vi "Report_Broken_VI.vi"(7 "before build?":bool=TRUE, 8 "error in (no error)":errorcluster, 10 "vi path":path, 11 "Build in":refnum<class "AB_Build.lvclass">) -> (0 "error out":errorcluster, 3 "Build out":refnum<class "AB_Build.lvclass">)   [LabVIEW 2020, in "AB_Build.lvclass"]
uses:
  <vilib>/AppBuilder/AB_Classes/Build/AB_Build.lvclass
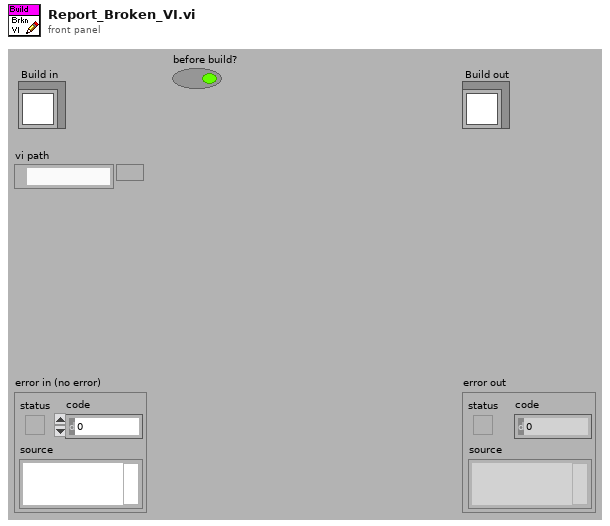
[diagram p1: front panel]
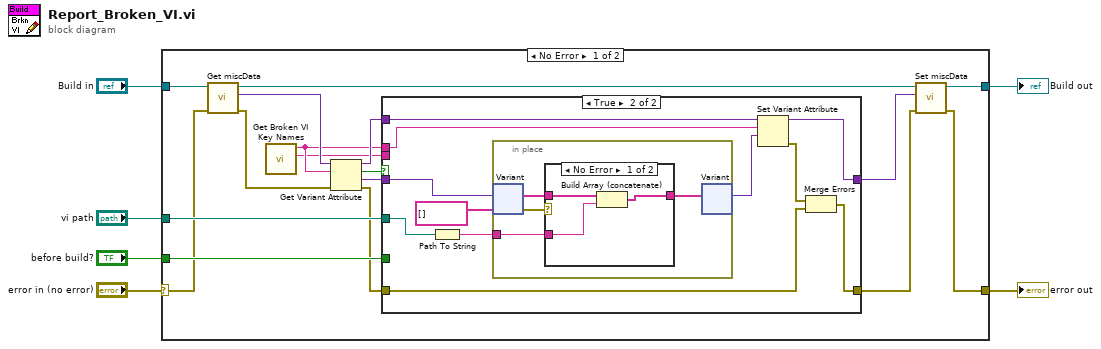
[diagram p0: block diagram]
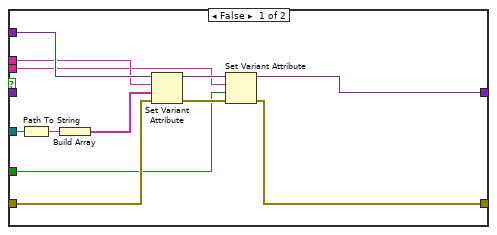
[diagram p2: hidden frame]
diagram:
  n1 = case shown="No Error" "error in (no error)" {
    selector: "error in (no error)" -> [w18 w56]
    tunnel: "Build in" -> [w23 w55]
    tunnel: [w21 w55] -> w5
    tunnel: [w11 w56] -> w4
    tunnel: "vi path" -> [w20 _]
    tunnel: "before build?" -> [w19 _]
    frame No Error {
      n2 = call-dynamic "Get miscData.vi"("error in (no error)"=w18, "AB_Build in"=w23) -> ("error out"=w15:errorcluster, "eng_miscData"=w17:variant, "AB_Build out"=w22:refnum<class "AB_Build.lvclass">)  [unwired: 7 in]
      n3 = call <vilib>:"Get Broken VI Key Names.vi"() -> ("Before Build Key"=w7:string, "Broken VIs List Key"=w8:string)  [unwired: 10 in]
      n4 = Get Variant Attribute(Variant=w17, name=w8, error in=w15) -> (duplicate Variant=w9:variant, found=w16:bool, value=w10:variant, error out=w13:errorcluster)  [unwired: 1 in]
      n5 = case shown="True" w16 {
        tunnel: w20 -> [w34 w46]
        tunnel: w19 -> [w27 _]
        tunnel: [w29 w38] -> w14
        tunnel: [w30 w42] -> w12
        tunnel: w13 -> [w31 w43]
        tunnel: w10 -> [_ w41]
        tunnel: w9 -> [w26 w39]
        tunnel: w8 -> [w25 w36]
        tunnel: w7 -> [w24 _]
        frame False {
          n6 = Path To String(path=w34) -> (string=w33:string)
          n7 = Build Array(w33) -> (w28:string[])
          n8 = Set Variant Attribute(Variant=w26, name=w25, value=w28, error in=w31) -> (Variant out=w35:variant, error out=w32:errorcluster)  [unwired: 1 out]
          n9 = Set Variant Attribute(Variant=w35, name=w24, value=w27, error in=w32) -> (Variant out=w29:variant, error out=w30:errorcluster)  [unwired: 1 out]
        }
        frame True {
          n10 = Path To String(path=w46) -> (string=w44:string)
          n11 = in-place {
            in-place-border: w44 -> [w50]
            n12 = in-place-variant #1(w41, string[] []) -> (w49:string[], w47:errorcluster)
            n13 = case shown="No Error" w47 {
              tunnel: w50 -> [w52 _]
              tunnel: w49 -> [w53 w54]
              tunnel: [w51 w54] -> w48
              frame No Error {
                n14 = Build Array (concatenate)(w53, w52) -> (w51:string[])
              }
              frame Error {
              }
            }
            n15 = in-place-variant #1(w48) -> (w40:variant)  [unwired: 1 out]
          }
          n16 = Set Variant Attribute(Variant=w39, name=w36, value=w40) -> (Variant out=w38:variant, error out=w37:errorcluster)  [unwired: 1 in, 1 out]
          n17 = Merge Errors(w37, w43) -> (w42:errorcluster)
        }
      }
      n18 = call-dynamic "Set miscData.vi"("error in (no error)"=w12, "eng_miscData"=w14, "AB_Build in"=w22) -> ("error out"=w11:errorcluster, "AB_Build out"=w21:refnum<class "AB_Build.lvclass">)  [unwired: 7 in]
    }
    frame Error {
    }
  }
  "error out" <- w4
  "Build out" <- w5
